vi "Choreo_TrajectorySwerve_GetSplit.vi"(9 "SplitIndex":i32, 11 "ChoreoTrajectorySwerve":T1) -> (3 "SplitSwerveTrajectory":T1)   [LabVIEW 2019, in "ChoreoLib.lvlib"]
doc: "Returns a choreo trajectory that represents the split of the trajectory at the given index.\n \nInputs: \n -- ChoreoTrajectorySwerve - cluster - data cluster for this trajectory \n -- splitIndex - integer - the index of the split trajectory to return.\n\nOutputs: \n -- SplitSwerveTrajectory - cluster - a choreo trajectory that represents the split of the trajectory at the given index."
uses:
  ChoreoLib.lvlib
  TypeDef/ChoreoTrajectorySwerve.ctl
  TypeDef/ChoreoSwerveSample.ctl
  TypeDef/ChoreoEventMarker.ctl
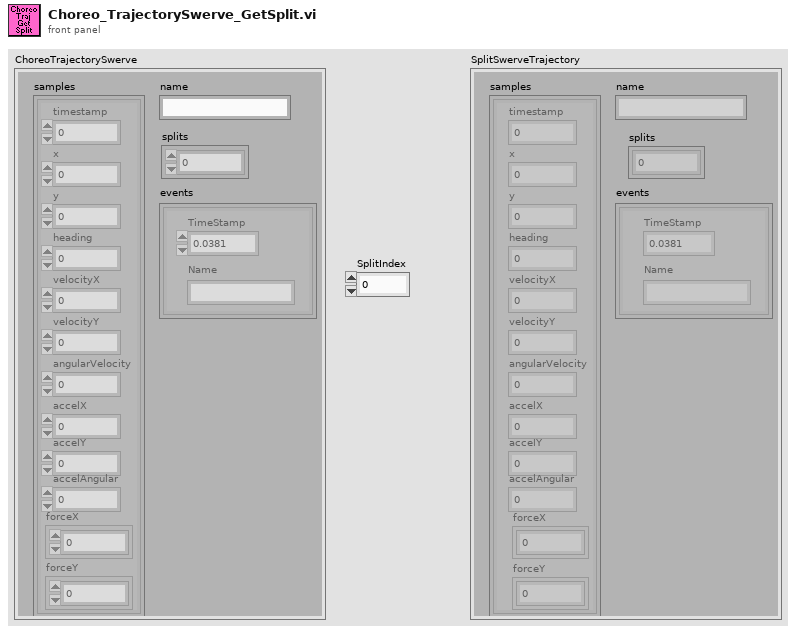
[diagram p1: front panel]
types:
  T1 = typedef "ChoreoLib.lvlib/ChoreoTrajectorySwerve.ctl" = cluster{"name":string, "samples":T2[], "splits":i32[], "events":T3[]}
  T2 = typedef "ChoreoLib.lvlib/ChoreoSwerveSample.ctl" = cluster{"timestamp":dbl, "x":dbl, "y":dbl, "heading":dbl, "velocityX":dbl, "velocityY":dbl, "angularVelocity":dbl, "accelX":dbl, "accelY":dbl, "accelAngular":dbl, "forceX":dbl[], "forceY":dbl[]}
  T3 = typedef "ChoreoLib.lvlib/ChoreoEventMarker.ctl" = cluster{"TimeStamp":dbl, "Name":string}
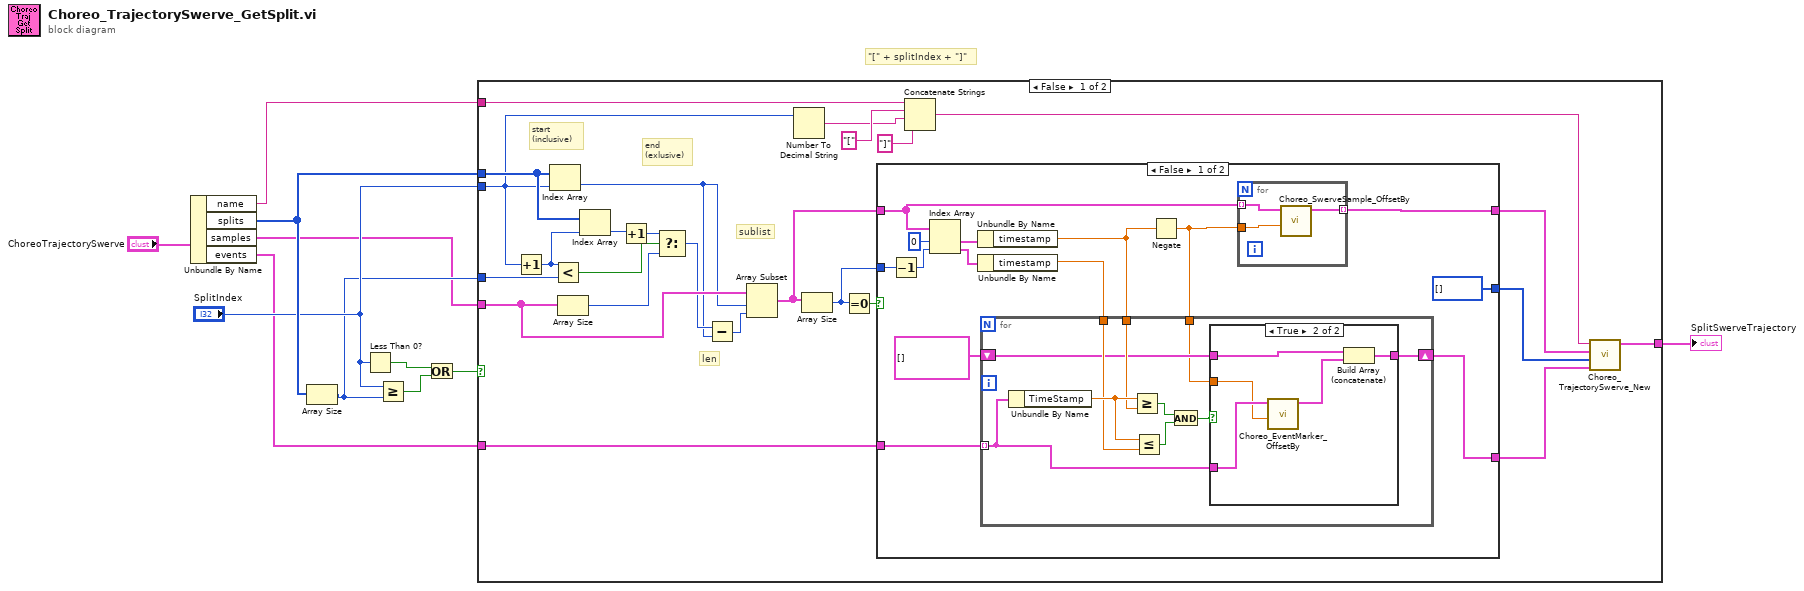
[diagram p0: block diagram]
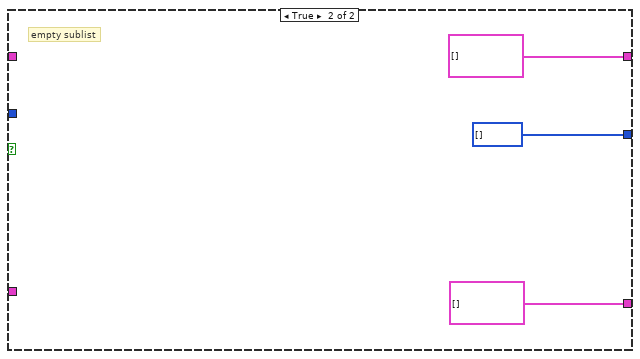
[diagram p3: hidden frame]
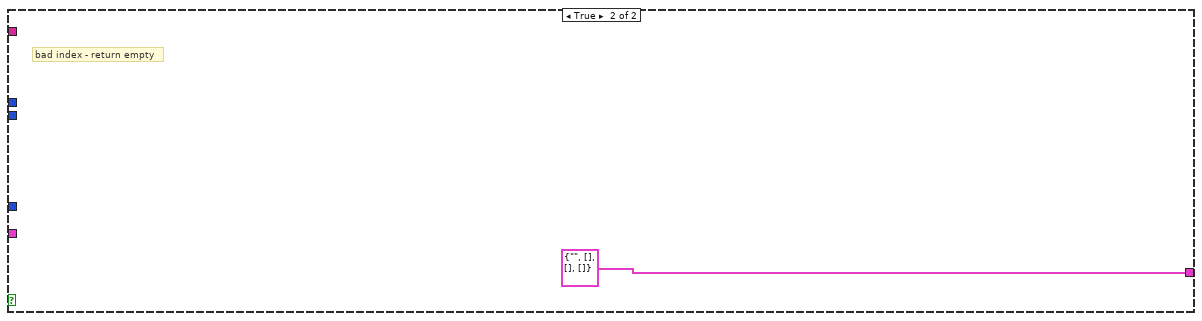
[diagram p4: hidden frame]
diagram:
  # "\"[\" + splitIndex + \"]\""
  n1 = Unbundle By Name("ChoreoTrajectorySwerve") -> ("name"=w2:string, "splits"=w6:i32[], "samples"=w3:T2[], "events"=w1:T3[])
  n2 = Array Size(array=w6) -> (size(s)=w4:i32)
  n3 = Less Than 0?(x="SplitIndex") -> (x < 0?=w10:bool)
  n4 = Greater Or Equal?(x="SplitIndex", y=w4) -> (x >= y?=w9:bool)
  n5 = Or(x=w10, y=w9) -> (x .or. y?=w8:bool)
  n6 = case shown="False" w8 {
    tunnel: [w24 T1 {"name"="", "samples"=[], "splits"=[], "events"=[]} ("ChoreoTrajectorySwerve")] -> w7
    tunnel: w6 -> [w35 _]
    tunnel: "SplitIndex" -> [w20 _]
    tunnel: w4 -> [w36 _]
    tunnel: w3 -> [w29 _]
    tunnel: w2 -> [w23 _]
    tunnel: w1 -> [w12 _]
    frame False {
      # "sublist"
      # "len"
      # "end\n(exlusive)"
      # "start \n(inclusive)"
      n7 = Increment(x=w20) -> (x+1=w34:i32)
      n8 = Index Array(array=w35, index=w20) -> (element=w27:i32)
      n9 = Less?(x=w34, y=w36) -> (x < y?=w31:bool)
      n10 = Array Size(array=w29) -> (size(s)=w30:i32)
      n11 = Index Array(array=w35, index=w34) -> (element=w33:i32)
      n12 = Increment(x=w33) -> (x+1=w32:i32)
      n13 = Select(t=w32, s=w31, f=w30) -> (s? t:f=w28:i32)
      n14 = Subtract(x=w28, y=w27) -> (x-y=w26:i32)
      n15 = Array Subset(array=w29, index=w27, length=w26) -> (w14:T2[])
      n16 = Number To Decimal String(number=w20) -> (decimal integer string=w19:string)  [unwired: 1 in]
      n17 = Array Size(array=w14) -> (size(s)=w13:i32)
      n18 = Equal To 0?(x=w13) -> (x = 0?=w25:bool)
      n19 = case shown="False" w25 {
        tunnel: [w44 T2[] [] ("samples")] -> w17
        tunnel: [i32[] [] ("splits") i32[] [] ("splits")] -> w16
        tunnel: [w38 T3[] [] ("events")] -> w15
        tunnel: w14 -> [w45 _]
        tunnel: w13 -> [w48 _]
        tunnel: w12 -> [w42 _]
        frame False {
          n20 = Decrement(x=w48) -> (x-1=w49:i32)
          n21 = Index Array(array=w45, index #1=0 ("index"), index #2=w49) -> (element #1=w47:T2, element #2=w46:T2)
          n22 = Unbundle By Name(w47) -> ("timestamp"=w41:dbl)
          n23 = Unbundle By Name(w46) -> ("timestamp"=w40:dbl)
          n24 = Negate(x=w41) -> (-x=w37:dbl)
          n25 = for {
            tunnel: w42 -> [w52] mode=indexing
            tunnel: w41 -> [w59]
            tunnel: w40 -> [w58]
            shift-right: [w53] -> w38
            shift-left: T3[] [] ("events") -> [w54]
            tunnel: w37 -> [w51]
            n26 = Unbundle By Name(w52) -> ("TimeStamp"=w60:dbl)
            n27 = Greater Or Equal?(x=w60, y=w59) -> (x >= y?=w57:bool)
            n28 = Less Or Equal?(x=w60, y=w58) -> (x <= y?=w56:bool)
            n29 = And(x=w57, y=w56) -> (x .and. y?=w55:bool)
            n30 = case shown="True" w55 {
              tunnel: w54 -> [w61 w66]
              tunnel: [w61 w65] -> w53
              tunnel: w52 -> [_ w64]
              tunnel: w51 -> [_ w63]
              frame False {
              }
              frame True {
                n31 = call "Choreo_EventMarker_OffsetBy.vi"("TimestampOffset"=w63, "EventMarker"=w64) -> ("offsetEventMarker"=w62:T3)  [unwired: 9 in]
                n32 = Build Array (concatenate)(w66, w62) -> (w65:T3[])
              }
            }
          }
          n33 = for {
            tunnel: w45 -> [w69] mode=indexing
            tunnel: w37 -> [w68]
            tunnel: [w67] -> w44 mode=indexing
            n34 = call "Choreo_SwerveSample_OffsetBy.vi"("TimeStampOffset"=w68, "ChoreoSwerveSample"=w69) -> ("OffsetSample"=w67:T2)  [unwired: 9 in]
          }
        }
        frame True {
          # "empty sublist"
        }
      }
      n35 = Concatenate Strings(w23, "[" ("string"), w19, "]" ("string")) -> (w18:string)
      n36 = call "Choreo_TrajectorySwerve_New.vi"("events"=w15, "splits"=w16, "samples"=w17, "name"=w18) -> ("ChoreoTrajectorySwerve"=w24:T1)  [unwired: 7 in]
    }
    frame True {
      # "bad index - return empty"
    }
  }
  "SplitSwerveTrajectory" <- w7
